vi "Write settings.vi"(7 "force saving?":bool, 8 "error in (no error)":errorcluster, 11 "ImagingModeSPIM in":refnum<class "ImagingModeSPIM.lvclass">) -> (0 "error out":errorcluster, 1 "cancelled":bool, 2 "settings name":string, 3 "ImagingModeSPIM out":refnum<class "ImagingModeSPIM.lvclass">)   [LabVIEW 2012, in "ImagingModeSPIM.lvclass"]
uses:
  ImagingModeSPIM.lvclass
  <vilib>/Distrio/Murmex/Murmex/Murmex.lvclass
  ImagingModeSPIM.lvclass/ImagingModeSPIM.ctl
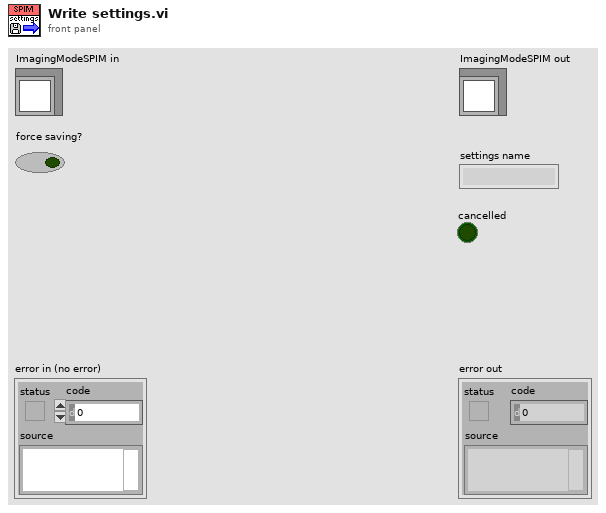
[diagram p1: front panel]
types:
  T1 = typedef "ImagingModeSPIM.lvclass/settings_cluster.ctl" = cluster{"Frequency":dbl[unit], "Waveform type":T2, "HSYNC pulses":i32, "y_resolution":i32, "line_exp":dbl[unit], "rolling_shutter":dbl[unit], "Waveform_data_fast":T3, "Waveform data galvo1":T3, "Waveform data galvo2":T3, "Pockels Cell":T4, "N_fast":dbl, "Staircase waveform":cluster{"Offset":dbl[unit], "step size":dbl[unit], "N_slow":dbl, "sampling info":cluster{"Fs":dbl, "#s":dbl}, "frequency_slow":dbl[unit], "Waveform type":T2}}
  T2 = typedef "ImagingModeSPIM.lvclass/waveform_enum.ctl" = enum16{"triangular", "step", "sawtooth", "sinusodial", "skewed sawtooth"}
  T3 = typedef "ImagingModeSPIM.lvclass/waveform data.ctl" = cluster{"Amplitude":dbl[unit], "Offset":dbl[unit], "Phase":dbl[unit], "Duty cycle":dbl, "sampling info":cluster{"Fs":dbl, "#s":dbl}, "frequency":dbl[unit], "Waveform type":T2}
  T4 = typedef "ImagingModeSPIM.lvclass/Pockels cell.ctl" = cluster{"Wavelength":T5, "digital ratio":dbl, "pulses per pixel":i32, "frequency":dbl[unit], "amplitude":dbl[unit], "phase":dbl[unit], "sampling info":cluster{"Fs":dbl, "#s":dbl}}
  T5 = typedef "ImagingModeSPIM.lvclass/wavelength_ring.ctl" = dbl
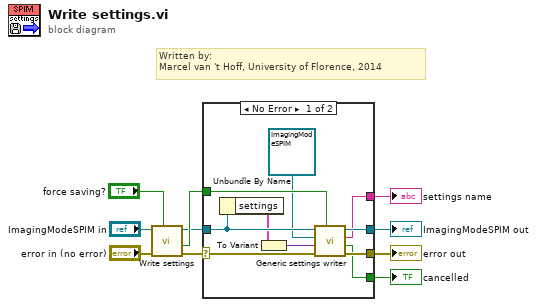
[diagram p0: block diagram]
diagram:
  # "Written by:\nMarcel van 't Hoff, University of Florence, 2014"
  n1 = call-parent "Write settings.vi"("force saving?"="force saving?", "error in (no error)"="error in (no error)", "Murmex in"="ImagingModeSPIM in") -> ("error out"=w7:errorcluster, "cancelled"=w6:bool, "Murmex out"=w5:refnum<class "ImagingModeSPIM.lvclass">)  [unwired: 5 in, 1 out]
  n2 = case shown="No Error" w7 {
    selector: w7 -> [w20 w22]
    tunnel: [w19 w22] -> w1
    tunnel: [w17 w21] -> w3
    tunnel: w5 -> [w18 w21]
    tunnel: [w16 _] -> w4
    tunnel: [w15 _] -> w2
    tunnel: w6 -> [w14 _]
    frame No Error {
      n3 = Unbundle By Name(w18) -> ("settings"=w13:T1)
      n4 = To Variant(anything=w13) -> (Variant=w12:variant)
      n5 = call <vilib>:"Generic settings writer.vi"("force saving?"=w14, "error in (no error)"=w20, "settings"=w12, "inheritance level"=refnum<class "ImagingModeSPIM.lvclass"> refnum ("ImagingModeSPIM"), "Murmex in"=w18) -> ("error out"=w19:errorcluster, "cancelled"=w15:bool, "settings name"=w16:string, "Murmex out"=w17:refnum<class "ImagingModeSPIM.lvclass">)  [unwired: 3 in]
    }
    frame Error {
    }
  }
  "error out" <- w1
  "ImagingModeSPIM out" <- w3
  "settings name" <- w4
  "cancelled" <- w2
